vi "DateTime (Set).vi"(6 "ISOBUS address":T3=-1 caption="ISOBUS address (-1)", 8 "error in":errorcluster, 10 "time stamp":timestamp, 11 "Mercury Reference In":T4) -> (0 "error out":errorcluster, 2 "Response":T2, 3 "Mercury Reference Out":T4, 4 "Valid?":T1)   [LabVIEW 2019, in "Mercury iXX.lvlib" / "System.lvlib"]
doc: "Set the date and time of the instrument to a date and time the user chooses."
uses:
  System.lvlib
  Controls/Mercury Reference.ctl
  CryoTUM_20210311/sub_vi-s/Equipment/Mercury iXX/Public/Controls/Comms Transport Layer.ctl
  Private/Controls/Query Dynamic Reference.ctl
  Controls/ISOBus Address.ctl
  Controls/Response String.ctl
  Controls/Is Valid LED.ctl
  mercury/Mercury iXX.lvlib
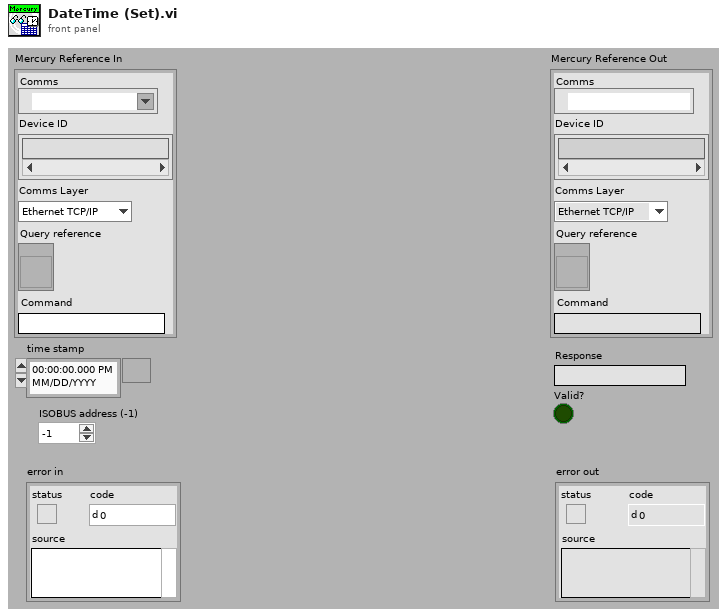
[diagram p1: front panel]
types:
  T1 = typedef "Mercury iXX.lvlib/Is Valid LED.ctl" = bool
  T2 = typedef "Mercury iXX.lvlib/Response String.ctl" = string
  T3 = typedef "Mercury iXX.lvlib/ISOBus Address.ctl" = i32
  T4 = typedef "Mercury iXX.lvlib/Mercury Reference.ctl" = cluster{"Comms":refnum<visa-resource-name>, "Device ID":string[], "Comms Layer":T5, "Command":string, "Query reference":T6}
  T5 = typedef "Mercury iXX.lvlib/Comms Transport Layer.ctl" = enum16{"Ethernet TCP/IP", "USB", "ISOBus - RS-232", "GPIB"}
  T6 = typedef "Mercury iXX.lvlib/Query Dynamic Reference.ctl" = refnum<vi>
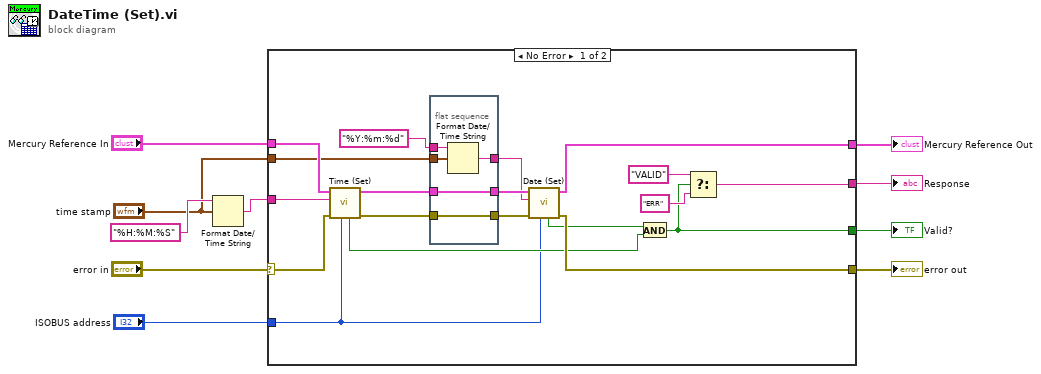
[diagram p0: block diagram]
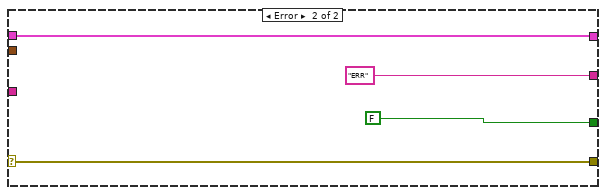
[diagram p2: hidden frame]
diagram:
  n1 = Format Date/Time String(time format string (%c)="%H:%M:%S", seconds (now)="time stamp") -> (date/time string=w4:string)  [unwired: 1 out]
  n2 = case shown="No Error" "error in" {
    selector: "error in" -> [w17 w37]
    tunnel: "Mercury Reference In" -> [w19 w38]
    tunnel: [w23 w38] -> w9
    tunnel: [w22 w37] -> w8
    tunnel: "ISOBUS address" -> [w13 _]
    tunnel: [w27 "ERR"] -> w5
    tunnel: w4 -> [w18 _]
    tunnel: [w26 FALSE] -> w3
    tunnel: "time stamp" -> [w11 _]
    frame No Error {
      n3 = call "Time (Set).vi"("ISOBUS address"=w13, "error in"=w17, "Time"=w18, "Mercury Reference In"=w19) -> ("error out"=w15:errorcluster, "Mercury Reference Out"=w14:T4, "Valid?"=w16:T1)  [unwired: 5 out]
      n4 = flat-sequence {
        tunnel: [w34] -> w24
        tunnel: "%Y:%m:%d" ("time format string (%c)") -> [w33]
        tunnel: w15 -> [w32]
        tunnel: [w32] -> w20
        tunnel: [w31] -> w25
        tunnel: w14 -> [w31]
        tunnel: w11 -> [w30]
        frame #0 {
          n5 = Format Date/Time String(time format string (%c)=w33, seconds (now)=w30) -> (date/time string=w34:string)  [unwired: 1 out]
        }
      }
      n6 = call "Date (Set).vi"("ISOBUS address"=w13, "error in"=w20, "Date"=w24, "Mercury Reference In"=w25) -> ("error out"=w22:errorcluster, "Mercury Reference Out"=w23:T4, "Valid?"=w21:T1)  [unwired: 5 out]
      n7 = And(x=w21, y=w16) -> (x .and. y?=w26:T1)
      n8 = Select(t="VALID" ("time format string (%c)"), s=w26, f="ERR" ("time format string (%c)")) -> (s? t:f=w27:string)
    }
    frame Error {
    }
  }
  "Mercury Reference Out" <- w9
  "error out" <- w8
  "Response" <- w5
  "Valid?" <- w3
